vi "Create Vacuum Test Page.vi"(7 "Data":string[][](array[string]), 8 "error in (no error)":errorcluster, 11 "Report In":refnum<class "NI_report.lvclass">) -> (0 "error out":errorcluster, 3 "Report Out":refnum<class "NI_report.lvclass">)   [LabVIEW 2014]
uses:
  <vilib>/Utility/NIReport.llb/NI_report.lvclass
  <vilib>/addons/_office/_exclsub.llb/font.ctl
  <vilib>/addons/_office/excel.llb/Excel Easy Table (str).vi
  <vilib>/addons/_office/NI_ReportGenerationToolkit.lvlib
  <vilib>/Utility/NIReport.llb/Excel/NI_Excel.lvclass
panel:
  in  "Start Cell":cluster{"row":i32, "column":i32}={"row"=3, "column"=0}
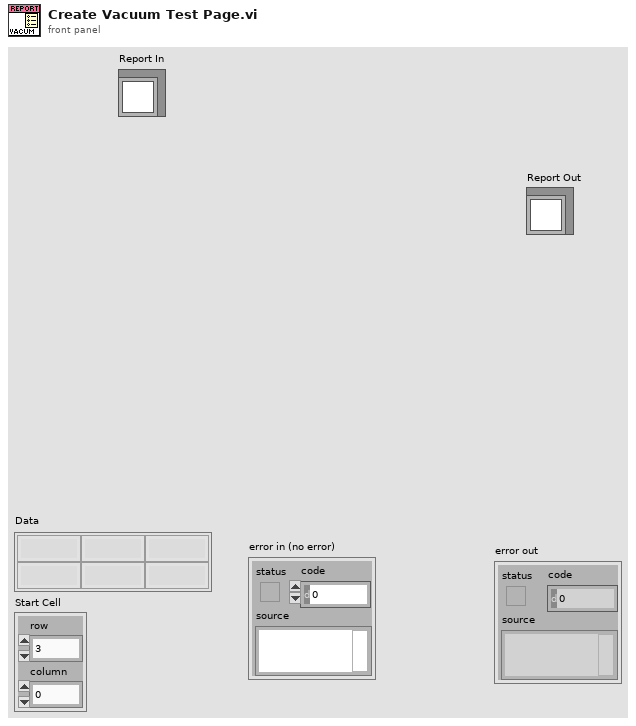
[diagram p1: front panel]
types:
  T1 = typedef "NI_ReportGenerationToolkit.lvlib/font.ctl" = cluster{"font name":string, "font size":dbl, "bold":u16, "italic":u16, "underline":u16, "strike through":u16, "font color":u32}
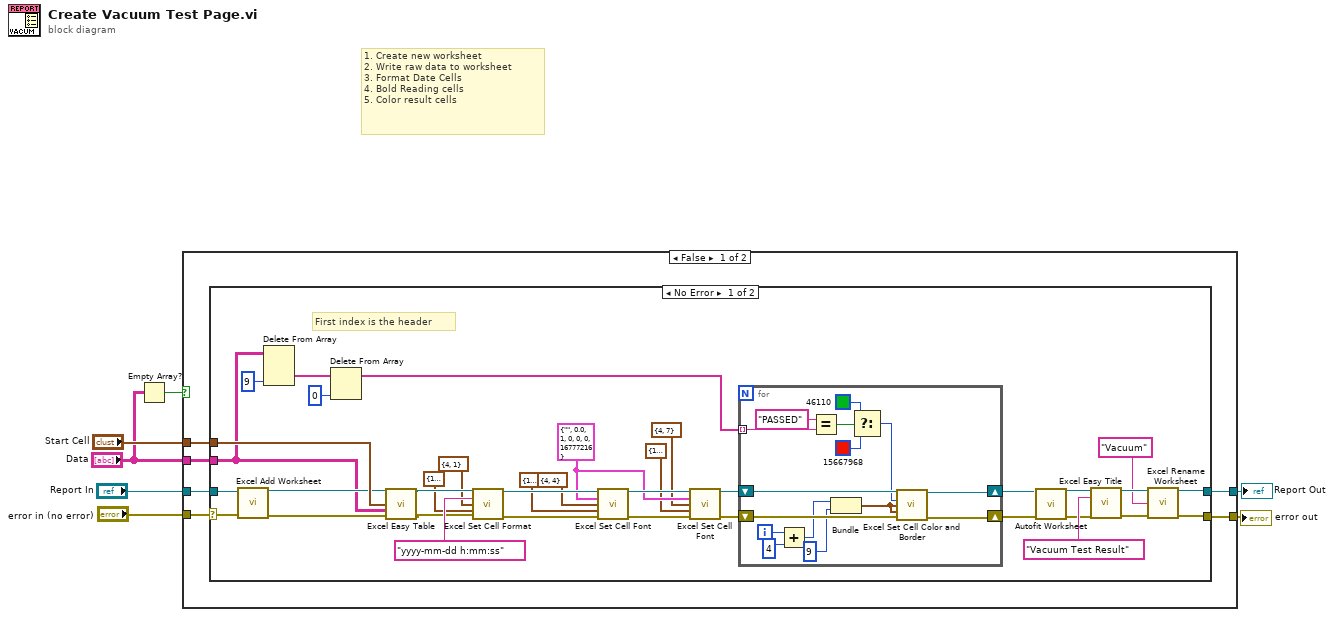
[diagram p0: block diagram]
diagram:
  # "1. Create new worksheet\n2. Write raw data to worksheet\n3. Format Date Cells\n4. Bold Reading cells\n5. Color result cells"
  n1 = Empty Array?(array="Data") -> (empty?=w1:bool)
  n2 = case shown="False" w1 {
    tunnel: [w13 w67] -> w7
    tunnel: "error in (no error)" -> [w12 w67]
    tunnel: "Report In" -> [w11 w68]
    tunnel: [w10 w68] -> w4
    tunnel: "Start Cell" -> [w9 _]
    tunnel: "Data" -> [w8 _]
    frame False {
      n3 = case shown="No Error" w12 {
        selector: w12 -> [w44 w66]
        tunnel: [w15 w66] -> w13
        tunnel: w11 -> [w45 w65]
        tunnel: [w16 w65] -> w10
        tunnel: w9 -> [w46 _]
        tunnel: w8 -> [w27 _]
        frame No Error {
          w30 = T1 {"font name"="", "font size"=0.0, "bold"=1, "italic"=0, "underline"=0, "strike through"=0, "font color"=16777216} ("font")
          # "First index is the header"
          n4 = call <vilib>:"Excel Add Worksheet.vi"("report in"=w45, "error in (no error)"=w44) -> ("report out"=w43:refnum<class "NI_report.lvclass">, "error out"=w42:errorcluster)  [unwired: 12 in]
          n5 = Delete From Array(array=w27, index (col)=9 ("disabled index (col)")) -> (deleted portion=w25:string[])  [unwired: 2 in, 1 out]
          n6 = Delete From Array(array=w25, index=0) -> (array with subset deleted=w22:string[])  [unwired: 1 in, 1 out]
          n7 = call-poly <vilib>:"Excel Easy Table.vi"("report in"=w43, "start (0, 0)"=w46, "text data"=w27, "error in (no error)"=w42) -> ("report out"=w40:refnum<class "NI_report.lvclass">, "error out"=w39:errorcluster)  [unwired: 7 in, 3 out]
          n8 = call <vilib>:"Excel Set Cell Format.vi"("report in"=w40, "number format"="yyyy-mm-dd h:mm:ss", "start (-1, -1)"=cluster{"row":i32, "column":i32} {"row"=4, "column"=1}, "end (-1, -1)"=cluster{"row":i32, "column":i32} {"row"=100, "column"=2} ("start (-1, -1)"), "error in (no error)"=w39) -> ("report out"=w36:refnum<class "NI_report.lvclass">, "error out"=w35:errorcluster)  [unwired: 9 in]
          n9 = call <vilib>:"Excel Set Cell Font.vi"("report in"=w36, "font"=w30, "start (-1, -1)"=cluster{"row":i32, "column":i32} {"row"=4, "column"=4}, "end (-1, -1)"=cluster{"row":i32, "column":i32} {"row"=100, "column"=4} ("start (-1, -1)"), "error in (no error)"=w35) -> ("report out"=w32:refnum<class "NI_report.lvclass">, "error out"=w31:errorcluster)  [unwired: 9 in]
          n10 = call <vilib>:"Excel Set Cell Font.vi"("report in"=w32, "font"=w30, "start (-1, -1)"=cluster{"row":i32, "column":i32} {"row"=4, "column"=7}, "end (-1, -1)"=cluster{"row":i32, "column":i32} {"row"=100, "column"=7} ("start (-1, -1)"), "error in (no error)"=w31) -> ("report out"=w24:refnum<class "NI_report.lvclass">, "error out"=w23:errorcluster)  [unwired: 9 in]
          n11 = for {
            tunnel: w22 -> [w64] mode=indexing
            shift-right: [w50] -> w20
            shift-left: w24 -> [w59]
            shift-right: [w56] -> w19
            shift-left: w23 -> [w57]
            i -> [w55]
            n12 = Add(x=w55, y=4) -> (x+y=w53:i32)
            n13 = Equal?(x="PASSED", y=w64) -> (x = y?=w62:bool)
            n14 = Bundle(w53, "y"=9) -> (w51:cluster{i32, "y":i32})  [unwired: 1 in]
            n15 = Select(t=u32 46110, s=w62, f=u32 15667968) -> (s? t:f=w58:u32)
            n16 = call <vilib>:"Excel Set Cell Color and Border.vi"("report in"=w59, "background color (w)"=w58, "start (-1, -1)"=w51, "end (-1, -1)"=w51, "error in (no error)"=w57) -> ("report out"=w50:refnum<class "NI_report.lvclass">, "error out"=w56:errorcluster)  [unwired: 9 in]
          }
          n17 = call "Autofit Worksheet.vi"("error in (no error)"=w19, "Report In"=w20) -> ("error out"=w47:errorcluster, "Report Out"=w48:refnum<class "NI_report.lvclass">)  [unwired: 8 in]
          n18 = call <vilib>:"Excel Easy Title.vi"("report in"=w48, "title"="Vacuum Test Result", "error in (no error)"=w47) -> ("report out"=w17:refnum<class "NI_report.lvclass">, "error out"=w18:errorcluster)  [unwired: 10 in, 1 out]
          n19 = call <vilib>:"Excel Rename Worksheet.vi"("report in"=w17, "worksheet name (\"\")"="Vacuum" ("worksheet name (\"\")"), "error in (no error)"=w18) -> ("report out"=w16:refnum<class "NI_report.lvclass">, "error out"=w15:errorcluster)  [unwired: 11 in]
        }
        frame Error {
        }
      }
    }
    frame True {
    }
  }
  "error out" <- w7
  "Report Out" <- w4
